vi "SM Process Exception Transition.vi"(6 "Message Queue In":refnum<class "Delacor_lib_QMH_Message Queue.lvclass">, 7 "Exception State":T2=enum."Error - Waiting For Action", 8 "error in (no error)":errorcluster, 10 "Data":variant, 11 "Exception Transition":T1) -> (0 "error out":errorcluster, 2 "Exception":errorcluster, 3 "State":T2)   [LabVIEW 2022 SP3, in "StateMachine.lvlib" / "HSE-State-Machine.lvlib"]
doc: "If an error occurs, go to the \"Erroring\" state and send an update to the UI\n____\nHAMPEL SOFTWARE ENGINEERING v2.6.0 (2023-12-19 10:54)"
uses:
  HSE-State-Machine.lvlib
  SM_States.ctl
  <vilib>/Delacor/Delacor QMH/Libraries/Message Queue_class/Delacor_lib_QMH_Message Queue.lvclass
  SM_Transitions.ctl
panel:
  # "Connector Pane"
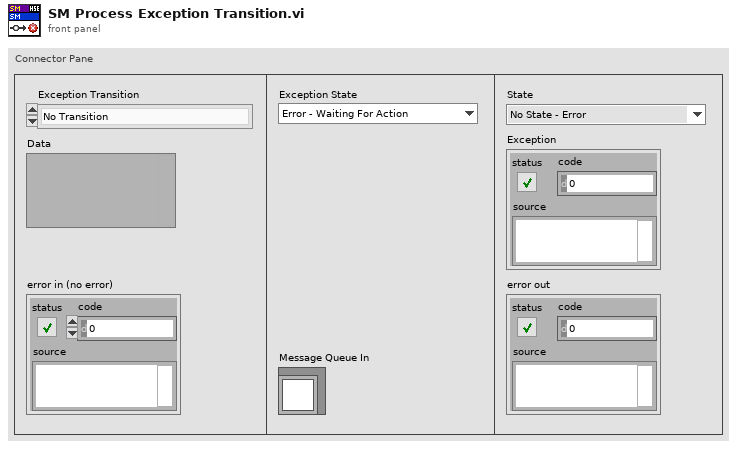
[diagram p1: front panel]
types:
  T1 = typedef "StateMachine.lvlib/HSE-State-Machine.lvlib/SM_Transitions.ctl" = enum16{"No Transition", "Exception", "Reset", "Initialization finished", "Process started", "Trigger detected", "Exit"}
  T2 = typedef "StateMachine.lvlib/HSE-State-Machine.lvlib/SM_States.ctl" = enum16{"No State - Error", "Error - Waiting For Action", "Initialising", "Standing by (idle)", "Waiting for External Trigger", "Polling for Signal Change", "Exiting"}
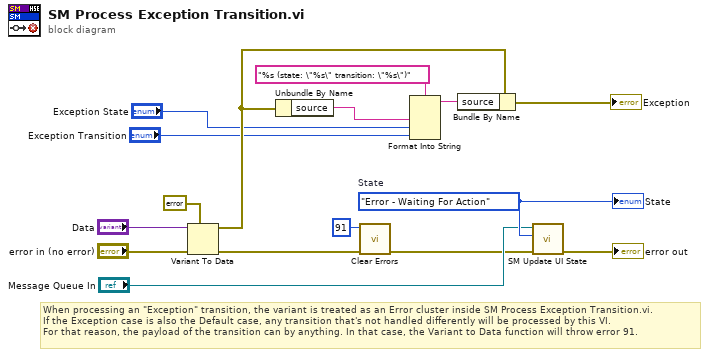
[diagram p0: block diagram]
diagram:
  w12 = SM_States."Error - Waiting For Action"  # State
  # "When processing an \"Exception\" transition, the variant is treated as an Error cluster inside SM Process Exception Transition.vi.\nIf the Exception case is also the Default case, any transition that's not handled differently will be processed by this VI. \nFor that reason, the payload of the transition can by anything. In that case, the Variant to Data function will throw error 91."
  n1 = Variant To Data(error in="error in (no error)", type=errorcluster {"status"=FALSE, "code"=0, "source"=""} ("error out"), Variant="Data") -> (data=w9:errorcluster, error out=w15:errorcluster)
  n2 = Unbundle By Name(w9) -> ("source"=w6:string)
  n3 = call <vilib>:"Clear Errors.vi"("error in (no error)"=w15, "specific error code to clear (0: all)"=91) -> ("error out"=w2:errorcluster)  [unwired: 4 in, 1 out]
  n4 = Format Into String(format string="%s (state: \"%s\" transition: \"%s\")", w6, "Exception State", "Exception Transition") -> (resulting string=w5:string)  [unwired: 2 in, 1 out]
  n5 = Bundle By Name(cluster=w9, "source"=w5) -> (→"Exception":errorcluster)
  n6 = call "SM Update UI State.vi"("error in (no error)"=w2, "State"=w12, "Message Queue In"="Message Queue In") -> ("error out"=→"error out":errorcluster)  [unwired: 7 in, 1 out]
  "State" <- w12
